vi "whileState.vi"(8 "error in (no error)":errorcluster, 11 "core in":refnum<class "core_state.lvclass">) -> (0 "error out":errorcluster, 1 "Done?":bool, 2 "next state":refnum<class "state.lvclass">, 3 "core out":refnum<class "core_state.lvclass">)   [LabVIEW 2020, in "eos.lvlib" / "core_state.lvclass"]
uses:
  core_state.lvclass
  C:/Projects/LVOS/EngineeringOS/source/interfaces/state/state.lvclass
  interfaces/state/state.lvclass
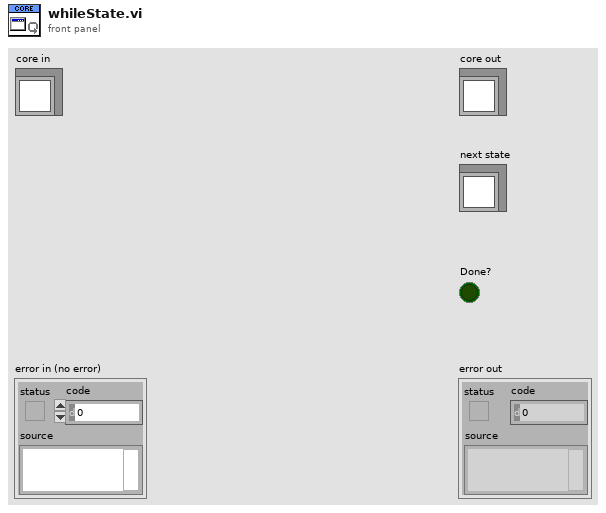
[diagram p1: front panel]
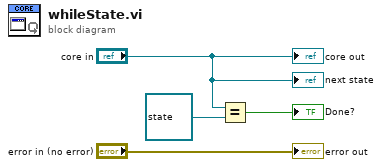
[diagram p0: block diagram]
diagram:
  n1 = Equal?(x="core in", y=refnum<class "state.lvclass"> refnum ("eos.lvlib:state.lvclass")) -> (x = y?=→"Done?":bool)
  "error out" <- "error in (no error)"
  "core out" <- "core in"
  "next state" <- "core in"
